vi "FW_Dead_Packet_for_Debug_170202.vi"() -> ()   [LabVIEW 2015]
panel:
  in  "Data to Send":u8[](array[numeric])=[0, 5, 4, 3, 0, 1, 0, 255, 255] format="%02x"
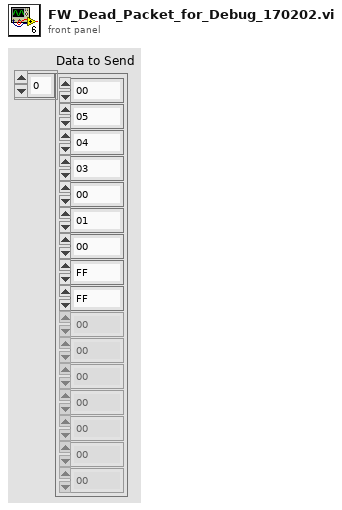
[diagram p1: front panel]
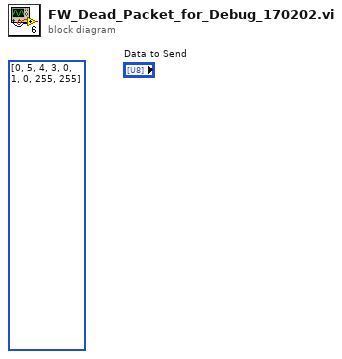
[diagram p0: block diagram]
diagram:
  (unwired) u8[] [0, 5, 4, 3, 0, 1, 0, 255, 255] ("Data to Send")
